vi "Modelloberfläche_Iod.vi"() -> ()   [LabVIEW 2018]
panel:
  in  "Anfangswerte (ne, nIm, nI2, nI, nIp, nI2p, te, tg) [m^-3] [K]":string="7.81363E17#1.15535E17#9.56487E18#1.75925E18#8.01418E17#9.54800E16#27551.44914#330.44553"
  in  "Anregungsenergie [eV]":dbl=9.5
  out "Fehlermeldung":string
  in  "Variation":string="40#50"
  out "standard output":string="40.0\r\n[6.21242824e+16 6.43700323e+16 2.95263983e+19 6.20032544e+19\r\n 6.42400539e+16 6.22542606e+16 2.96179006e+04 2.98683360e+02]\r\nne: 62124282374475656.000000\r\nnIm: 64370032268105840.000000\r\nnI2: 29526398259315437568.000000\r\nnI: 62003254385976975360.000000\r\nnIp: 64240053935001104.000000\r\nnI2p: 62254260581188208.000000\r\nte: 29617.900642\r\ntg: 298.683360\r\n34.72778878632954\r\n34.72778878632954\r\n14.120865931881333\r\n20.60692285444821\r\n0.06429551869940268\r\n50.0\r\n[7.75656064e+16 6.69909664e+16 2.55410441e+19 6.65464558e+19\r\n 8.05432147e+16 6.40133575e+16 2.93592908e+04 3.00193820e+02]\r\nne: 77565606381735856.000000\r\nnIm: 66990966414534968.000000\r\nnI2: 25541044121169461248.000000\r\nnI: 66546455777303076864.000000\r\nnIp: 80543214673077856.000000\r\nnI2p: 64013357459760424.000000\r\nte: 29359.290760\r\ntg: 300.193820\r\n40.12420492526585\r\n40.12420492526585\r\n14.436287991464793\r\n25.68791693380106\r\n0.07181354763631792\r\nLaufzeit:\r\n2.7240045070648193\r\n0.04540007511774699\r\n" caption="Standardausgabe"
  in  "Simulation starten":bool
  in  "Strom [mA]":dbl=100.0
  out "?":string="RF Leistung [W]"
  in  "Fluss [mg/s]":dbl=1.0
  in  "RF Leistung [W]":dbl=100.0
  in  "Was soll variiert werden?":bool=TRUE
  in  "Abstand Gitter [m]":dbl=0.001
  in  "Gitterspannung [V]":dbl=1500.0
  in  "Widerstand [Ohm]":dbl=0.975
  in  "Windungen":dbl=6.0
  in  "Frequenz [MHz]":dbl=1.1
  in  "Beta g":dbl=0.0976
  in  "Beta i":dbl=0.5
  in  "Länge [m]":dbl=0.055
  in  "Radius [m]":dbl=0.05
  in  "Variation oder Performancekurve ?":bool
  # "Iod"
  # "Variation"
  # "Performance"
  # "Fluss"
  # "RF Leistung"
  # "Variation von:"
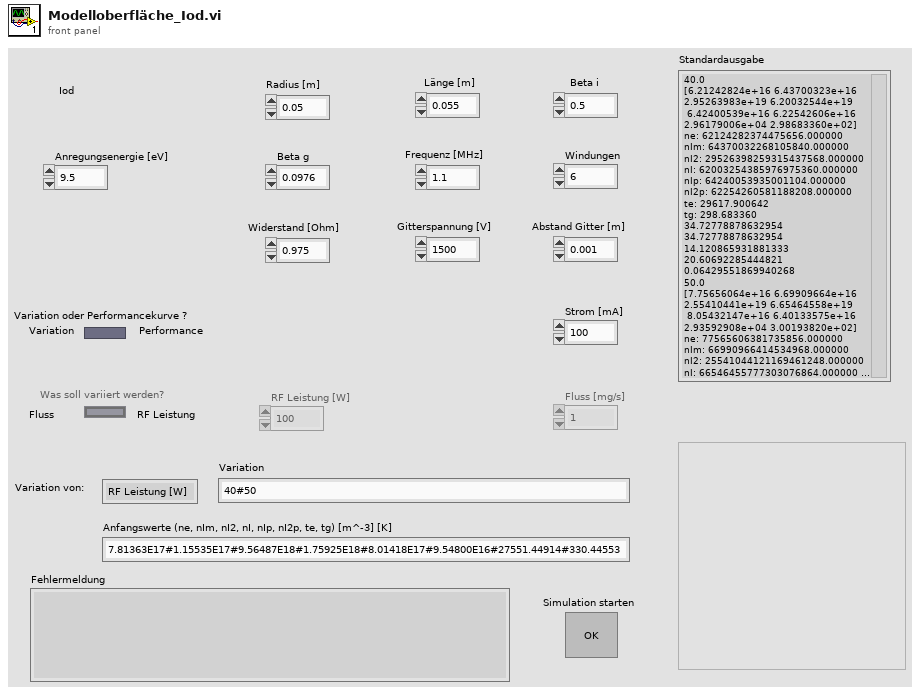
[diagram p1: front panel]
types:
  T1 = enum8{"Enabled", "Disabled", "Disabled and Grayed Out"}
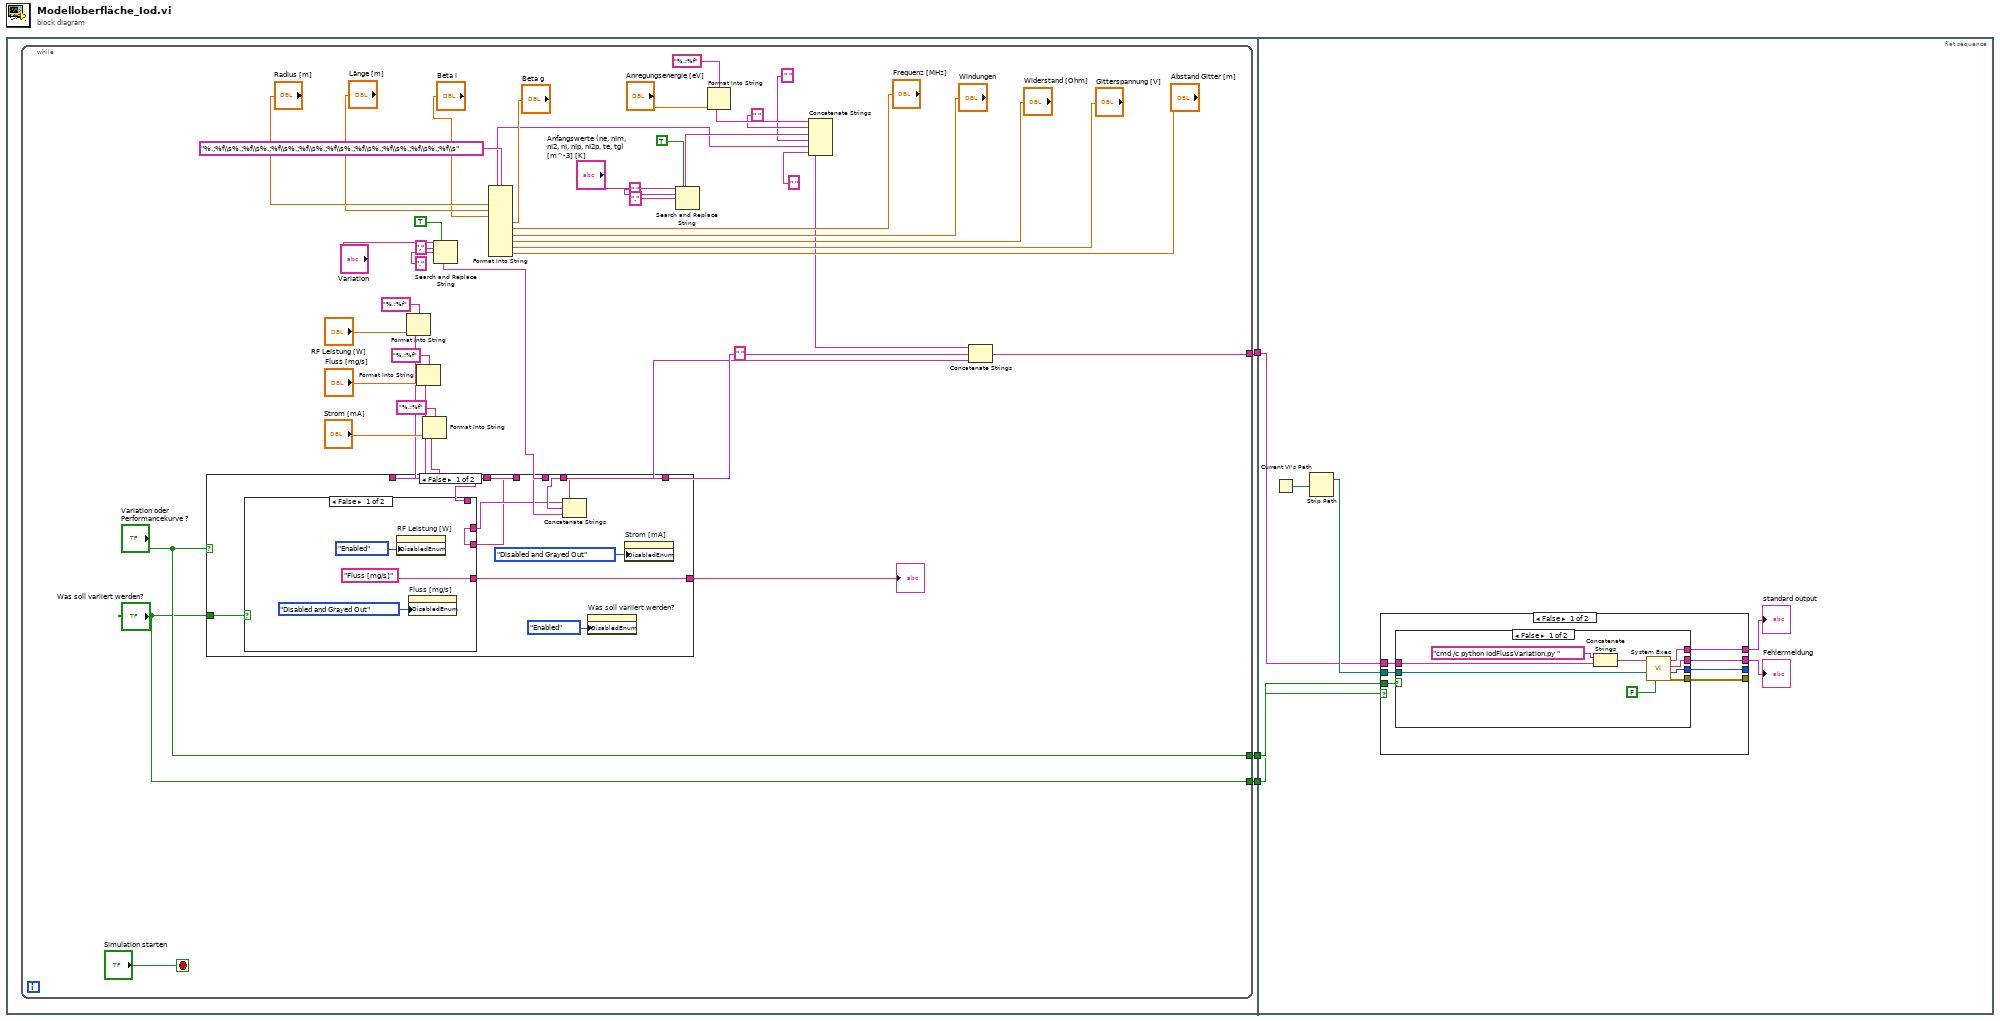
[diagram p0: block diagram]
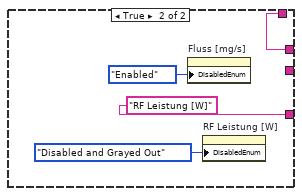
[diagram p2: hidden frame]
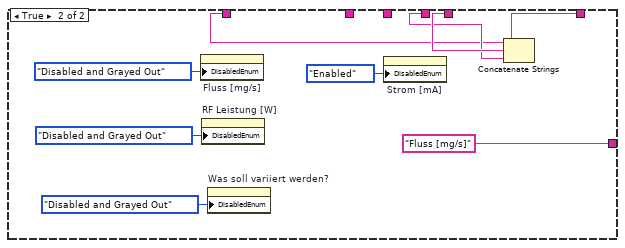
[diagram p3: hidden frame]
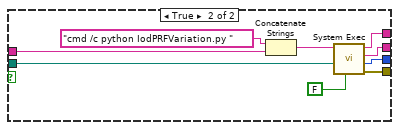
[diagram p4: hidden frame]
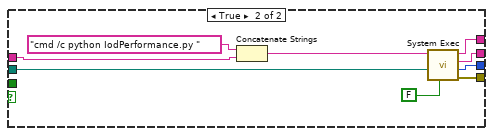
[diagram p5: hidden frame]
diagram:
  n1 = flat-sequence {
    tunnel: [w6] -> w3
    tunnel: [w5] -> w2
    tunnel: [w4] -> w1
    tunnel: w3 -> [w82]
    tunnel: w2 -> [w79]
    tunnel: w1 -> [w78]
    frame #0 {
      n2 = while {
        tunnel: [w29] -> w6
        tunnel: ["Variation oder Performancekurve ?"] -> w5
        tunnel: ["Was soll variiert werden?"] -> w4
        stop <- "Simulation starten" stop-if-true
        w30 = " "
        n3 = Format Into String(format string="%.;%f" ("Format-String"), "RF Leistung [W]") -> (resulting string=w27:string)  [unwired: 2 in, 1 out]
        n4 = Format Into String(format string="%.;%f" ("Format-String"), "Fluss [mg/s]") -> (resulting string=w31:string)  [unwired: 2 in, 1 out]
        n5 = Format Into String(format string="%.;%f" ("Format-String"), "Strom [mA]") -> (resulting string=w32:string)  [unwired: 2 in, 1 out]
        n6 = Search and Replace String(replace all?=TRUE ("Alle ersetzen? (F)"), input string="Variation", search string="," ("Such-String"), replace string="." ("Ersetzungs-String (\"\")")) -> (result string=w25:string)  [unwired: 4 in, 3 out]
        n7 = case shown="False" "Variation oder Performancekurve ?" {
          tunnel: "Was soll variiert werden?" -> [w60 _]
          tunnel: [w57 "Fluss [mg/s]"] -> w39
          tunnel: w25 -> [w54 w71]
          tunnel: [w56 w70] -> w28
          tunnel: w32 -> [_ w69]
          tunnel: w31 -> [w51 _]
          tunnel: w27 -> [w52 _]
          tunnel: w30 -> [w55 w72]
          frame False {
            n8 = case shown="False" w60 {
              tunnel: ["Fluss [mg/s]" "RF Leistung [W]"] -> w57
              tunnel: w51 -> [_ w65]
              tunnel: [w61 w65] -> w53
              tunnel: w52 -> [w61 _]
              frame False {
                n9 = property on="RF Leistung [W]" class="DigWert (strikt)"("DisabledEnum"=T1."Enabled" ("Deaktiviert")) -> ()  [unwired: 2 in, 2 out]
                n10 = property on="Fluss [mg/s]" class="DigWert (strikt)"("DisabledEnum"=T1."Disabled and Grayed Out" ("Deaktiviert")) -> ()  [unwired: 2 in, 2 out]
              }
              frame True {
                n11 = property on="Fluss [mg/s]" class="DigWert (strikt)"("DisabledEnum"=T1."Enabled" ("Deaktiviert")) -> ()  [unwired: 2 in, 2 out]
                n12 = property on="RF Leistung [W]" class="DigWert (strikt)"("DisabledEnum"=T1."Disabled and Grayed Out" ("Deaktiviert")) -> ()  [unwired: 2 in, 2 out]
              }
            }
            n13 = Concatenate Strings(w53, w55, w54) -> (w56:string)
            n14 = property on="Was soll variiert werden?" class="Bool. (strikt)"("DisabledEnum"=T1."Enabled" ("Deaktiviert")) -> ()  [unwired: 2 in, 2 out]
            n15 = property on="Strom [mA]" class="DigWert (strikt)"("DisabledEnum"=T1."Disabled and Grayed Out" ("Deaktiviert")) -> ()  [unwired: 2 in, 2 out]
          }
          frame True {
            n16 = property on="Fluss [mg/s]" class="DigWert (strikt)"("DisabledEnum"=T1."Disabled and Grayed Out" ("Deaktiviert")) -> ()  [unwired: 2 in, 2 out]
            n17 = property on="RF Leistung [W]" class="DigWert (strikt)"("DisabledEnum"=T1."Disabled and Grayed Out" ("Deaktiviert")) -> ()  [unwired: 2 in, 2 out]
            n18 = property on="Was soll variiert werden?" class="Bool. (strikt)"("DisabledEnum"=T1."Disabled and Grayed Out" ("Deaktiviert")) -> ()  [unwired: 2 in, 2 out]
            n19 = property on="Strom [mA]" class="DigWert (strikt)"("DisabledEnum"=T1."Enabled" ("Deaktiviert")) -> ()  [unwired: 2 in, 2 out]
            n20 = Concatenate Strings(w69, w72, w71) -> (w70:string)
          }
        }
        "?" <- w39
        n21 = Format Into String(format string="%.;%f\\s%.;%f\\s%.;%f\\s%.;%f\\s%.;%f\\s%.;%f\\s%.;%f\\s%.;%f\\s%.;%f\\s" ("Format-String"), "Radius [m]", "Länge [m]", "Beta i", "Beta g", "Frequenz [MHz]", "Windungen", "Widerstand [Ohm]", "Gitterspannung [V]", "Abstand Gitter [m]") -> (resulting string=w8:string)  [unwired: 2 in, 1 out]
        n22 = Search and Replace String(replace all?=TRUE ("Alle ersetzen? (F)"), input string="Anfangswerte (ne, nIm, nI2, nI, nIp, nI2p, te, tg) [m^-3] [K]", search string="." ("Such-String"), replace string="." ("Ersetzungs-String (\"\")")) -> (result string=w10:string)  [unwired: 4 in, 3 out]
        n23 = Format Into String(format string="%.;%f" ("Format-String"), "Anregungsenergie [eV]") -> (resulting string=w12:string)  [unwired: 2 in, 1 out]
        n24 = Concatenate Strings(w12, " " ("String"), w10, " " ("String"), w8, " " ("String")) -> (w15:string)
        n25 = Concatenate Strings(w15, w30, w28) -> (w29:string)
      }
    }
    frame #1 {
      n26 = Current VI's Path() -> (path=w84:path)
      n27 = Strip Path(path=w84) -> (stripped path=w83:path)  [unwired: 1 out]
      n28 = case shown="False" w79 {
        tunnel: w82 -> [w91 w115]
        tunnel: [w90 w114] -> _
        tunnel: [w89 w113] -> _
        tunnel: [w88 w112] -> w80
        tunnel: [w87 w111] -> w81
        tunnel: w83 -> [w86 w110]
        tunnel: w78 -> [w85 _]
        frame False {
          n29 = case shown="False" w85 {
            tunnel: w91 -> [w97 w106]
            tunnel: [w96 w105] -> w90
            tunnel: [w95 w104] -> w89
            tunnel: [w94 w103] -> w88
            tunnel: [w93 w102] -> w87
            tunnel: w86 -> [w92 w101]
            frame False {
              n30 = Concatenate Strings("cmd /c python IodFlussVariation.py " ("String"), w97) -> (w100:string)
              n31 = call <vilib>:"System Exec.vi"("run minimized? (F)"=FALSE, "working directory"=w92, "command line"=w100) -> ("error out"=w96:errorcluster, "return code"=w95:i32, "standard error"=w94:string, "standard output"=w93:string)  [unwired: 5 in]
            }
            frame True {
              n32 = Concatenate Strings("cmd /c python IodPRFVariation.py " ("String"), w106) -> (w109:string)
              n33 = call <vilib>:"System Exec.vi"("run minimized? (F)"=FALSE, "working directory"=w101, "command line"=w109) -> ("error out"=w105:errorcluster, "return code"=w104:i32, "standard error"=w103:string, "standard output"=w102:string)  [unwired: 5 in]
            }
          }
        }
        frame True {
          n34 = Concatenate Strings("cmd /c python IodPerformance.py " ("String"), w115) -> (w118:string)
          n35 = call <vilib>:"System Exec.vi"("run minimized? (F)"=FALSE, "working directory"=w110, "command line"=w118) -> ("error out"=w114:errorcluster, "return code"=w113:i32, "standard error"=w112:string, "standard output"=w111:string)  [unwired: 5 in]
        }
      }
      "standard output" <- w81
      "Fehlermeldung" <- w80
    }
  }
